vi "Stop.vi"() -> ()   [LabVIEW 2012]
panel:
  in  "stop":bool
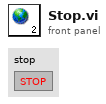
[diagram p1: front panel]
diagram:
